vi "Create File.vi"(8 "error in":errorcluster, 11 "XLS in":refnum<class "XLS.lvclass">) -> (0 "error out":errorcluster, 3 "XLS out":refnum<class "XLS.lvclass">)   [LabVIEW 2017, in "Report_lib.lvlib" / "XLS.lvclass"]
doc: "This method create XLS document based on local Template\nand setup font and text properties"
uses:
  XLS.lvclass
  XLS.lvclass/XLS.ctl
  <vilib>/Utility/NIReport.llb/NI_report.lvclass
  <vilib>/Utility/NIReport.llb/Excel/NI_Excel.lvclass
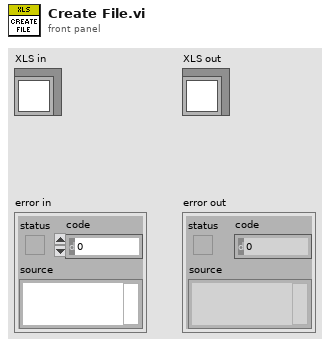
[diagram p1: front panel]
types:
  T1 = enum16{"maximized", "minimized", "normal", "no change"}
  T2 = enum16{"Standard Report", "HTML", "Word", "Excel"}
  T3 = cluster{"Charset (-1)":i16, "Weight (-1)":i16, "Name":string, "Size":string}
  T4 = cluster{"Italic":enum16{"Italic Unchanged", "Italic On", "Italic Off"}, "Strike Through":enum16{"Strike Through Unchanged", "Strike Through On", "Strike Through Off"}, "Underline":enum16{"Underline Unchanged", "Underline On", "Underline Off"}, "Bold":enum16{"Bold Unchanged", "Bold On", "Bold Off"}}
  T5 = enum32{"invalid app kind", "Development System", "Run Time System", "Student Edition", "Embedded LabVIEW", "Evaluation", "Custom"}
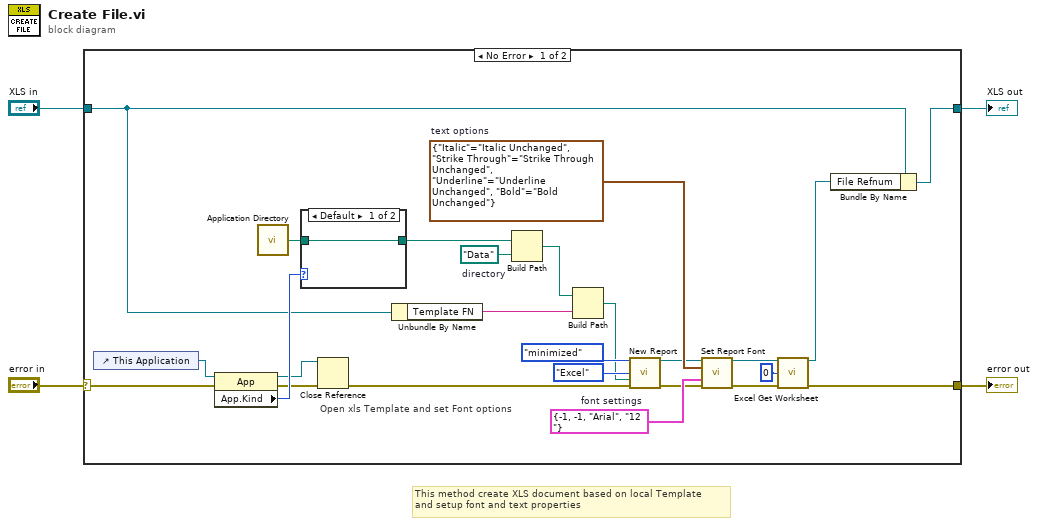
[diagram p0: block diagram]
diagram:
  # "This method create XLS document based on local Template\nand setup font and text properties"
  n1 = case shown="No Error" "error in" {
    selector: "error in" -> [w13 w33]
    tunnel: [w10 w33] -> w3
    tunnel: [w12 w32] -> w1
    tunnel: "XLS in" -> [w6 w32]
    frame No Error {
      w22 = path "Data"  # directory
      w29 = T3 {"Charset (-1)"=-1, "Weight (-1)"=-1, "Name"="Arial", "Size"="12 "}  # font settings
      w28 = T4 {"Italic"=enum."Italic Unchanged", "Strike Through"=enum."Strike Through Unchanged", "Underline"=enum."Underline Unchanged", "Bold"=enum."Bold Unchanged"}  # text options
      # "Open xls Template and set Font options"
      n2 = control-ref of="This Application"() -> (w9:refnum<vi>)
      n3 = property class="App"(reference=w9, error in=w13) -> (reference out=w15:refnum<vi>, error out=w16:errorcluster, "App.Kind"=w17:T5)
      n4 = call <vilib>:"Application Directory.vi"() -> ("Application Directory"=w8:path)
      n5 = case shown="Default" w17 {
        tunnel: w8 -> [w30 w31]
        tunnel: [w30 w31] -> w7
        frame Default {
        }
        frame "Run Time System" {
        }
      }
      n6 = Close Reference(reference=w15, error in (no error)=w16) -> (error out=w14:errorcluster)
      n7 = Unbundle By Name(w6) -> ("Template FN"=w5:string)
      n8 = Build Path(base path=w7, name or relative path=w22) -> (appended path=w21:path)
      n9 = Build Path(base path=w21, name or relative path=w5) -> (appended path=w23:path)
      n10 = call <vilib>:"New Report.vi"("window state (normal)"=T1."minimized", "report type"=T2."Excel", "template (empty)"=w23, "error in (no error)"=w14) -> ("report out"=w26:refnum<class "NI_report.lvclass">, "error out"=w27:errorcluster)  [unwired: 10 in]
      n11 = call-dynamic "Set Report Font.vi"("report in"=w26, "text options"=w28, "font settings"=w29, "error in (no error)"=w27) -> ("report out"=w18:refnum<class "NI_report.lvclass">, "error out"=w19:errorcluster)  [unwired: 9 in, 1 out]
      n12 = call <vilib>:"Excel Get Worksheet.vi"("report in"=w18, "worksheet index (0)"=0, "error in (no error)"=w19) -> ("report out"=w11:refnum<class "NI_report.lvclass">, "error out"=w10:errorcluster)  [unwired: 11 in]
      n13 = Bundle By Name(cluster=w6, "File Refnum"=w11) -> (w12:refnum<class "XLS.lvclass">)
    }
    frame Error {
    }
  }
  "error out" <- w3
  "XLS out" <- w1
